vi "TDMS Logging Loop.vi"(6 "Logging Period (ms)":i64=20, 7 "Buffer Size":u32=1000, 9 "Group Initialization":T1(array[cluster]), 10 "TDMS Name":string="Test", 11 "Log to USB?":bool) -> ()   [LabVIEW 2015]
uses:
  <userlib>/836-Library/System/TDMSv2/Group Data.ctl
  <userlib>/836-Library/System/TDMSv2/Group Channels.ctl
  <vilib>/Platform/TimedLoop/XDataNode/timing_clust.ctl
  <vilib>/Platform/TimedLoop/XDataNode/nitl_modes.ctl
  <vilib>/Platform/TimedLoop/XDataNode/wakeup.ctl
  <userlib>/836-Library/System/TDMSv2/TDMS RT FIFO Packet.ctl
  <userlib>/836-Library/System/TDMSv2/Channel Initializer.ctl
  <userlib>/836-Library/System/TDMSv2/Back Channel Data.ctl
  <vilib>/platform/TimedLoop/XDataNode/XDataNode.xnode
  <vilib>/Platform/TimedLoop/XDataNode/XDNodeRunTimeDep.lvlib
panel:
  out "Cluster 2":T4
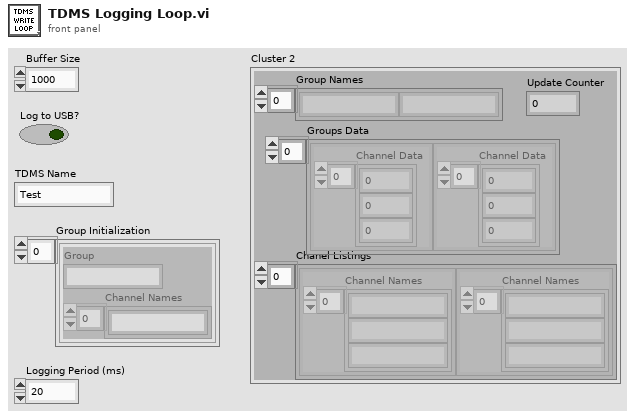
[diagram p1: front panel]
types:
  T1 = cluster{"Group":string, "Channel Names":string[]}[]
  T2 = typedef "Group Data.ctl" = cluster{"Channel Data":dbl[]}
  T3 = typedef "Group Channels.ctl" = cluster{"Channel Names":string[]}
  T4 = cluster{"Group Names":string[], "Groups Data":T2[], "Update Counter":i32, "Chanel Listings":T3[]}
  T5 = enum16{"open", "open or create", "create or replace", "create", "open (read-only)"}
  T6 = typedef "XDNodeRunTimeDep.lvlib/timing_clust.ctl" = cluster{"Expected End [f-1]":u64, "Actual End [f-1]":u64, "Finished Late? [f-1]":bool, "Expected End [i-1]":u64, "Actual End [i-1]":u64, "Finished Late? [i-1]":bool, "Expected Start [i]":u64, "Actual Start [i]":u64, "Expected Start [f]":u64, "Actual Start [f]":u64, "Source Name":string, "Structure Name":string, "Period":i64, "Deadline":i64, "Offset":i64, "Start":i64, "Priority":i32, "Timeout":i32, "Mode":T7, "Wakeup Reason":T8, "Error":errorcluster, "Source Type":string, "Secondary Source Type":string, "Global End Time":u64, "Global Start Time":u64, "Frame Duration":u64, "Iteration Duration":u64, "Assigned CPU":i32, "I/O Scan Engine Mode":u32}
  T7 = typedef "XDNodeRunTimeDep.lvlib/nitl_modes.ctl" = enum32{"No Change", "Process missed periods, maintain original phase", "Discard missed periods, maintain original phase", "Process missed periods, ignore original phase", "Discard missed periods, ignore original phase"}
  T8 = typedef "XDNodeRunTimeDep.lvlib/wakeup.ctl" = enum32{"Normal", "Aborted", "Asynchronous wakeup", "Timing source error", "Timed loop error", "Timeout"}
  T9 = typedef "Channel Initializer.ctl" = cluster{"Column Headers":string[], "Initialization array":dbl[]}
  T10 = typedef "TDMS RT FIFO Packet.ctl" = cluster{"Group/CMD":i32, "Data":dbl, "Channel":i32}
  T11 = typedef "Back Channel Data.ctl" = cluster{"Group":string, "Channel":string, "Return Notifier":refnum<notifier>}
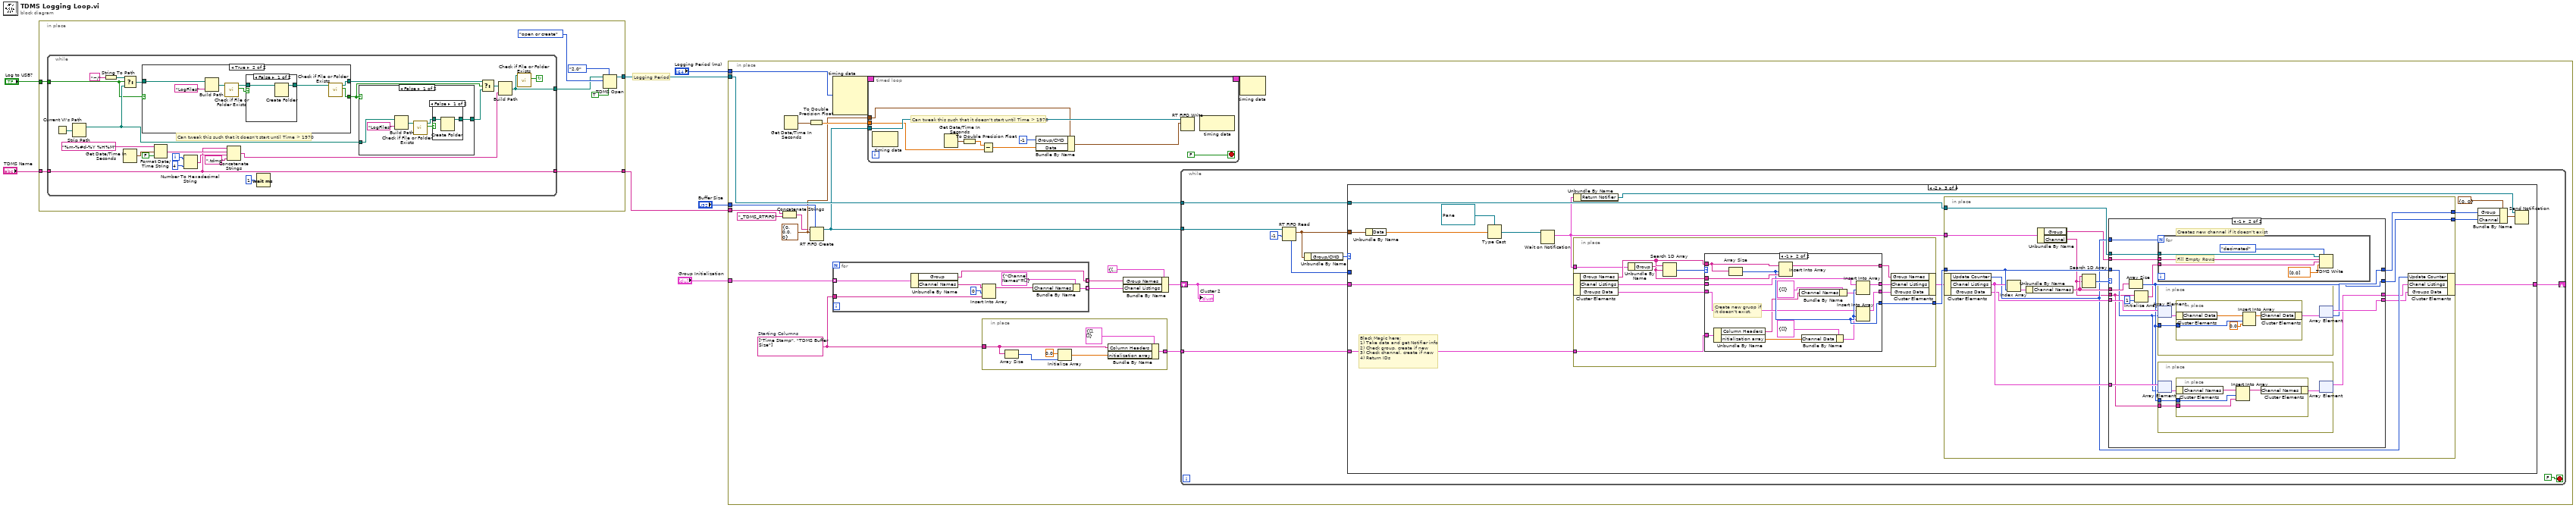
[diagram p0: block diagram]
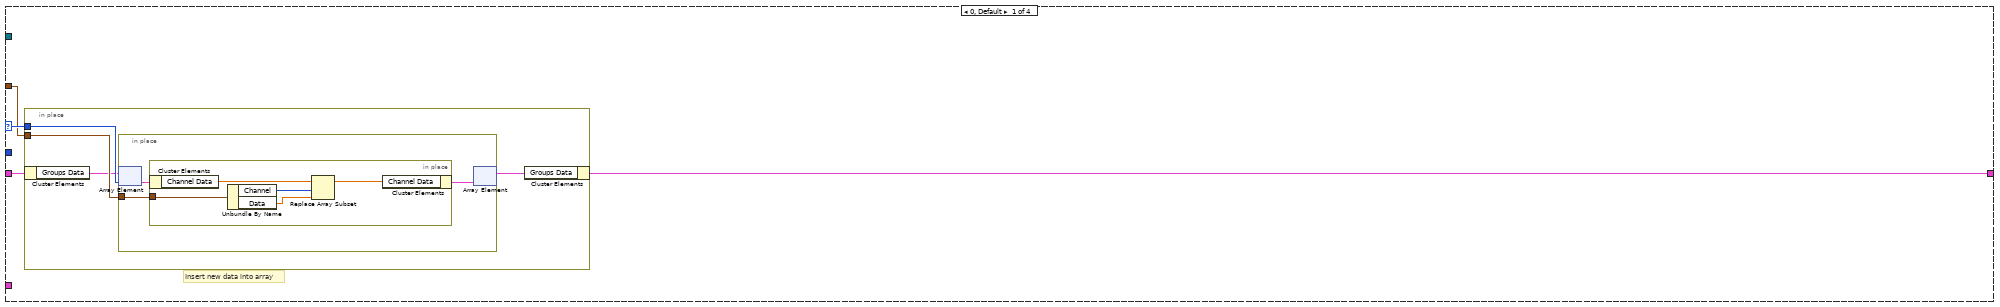
[diagram p6: hidden frame]
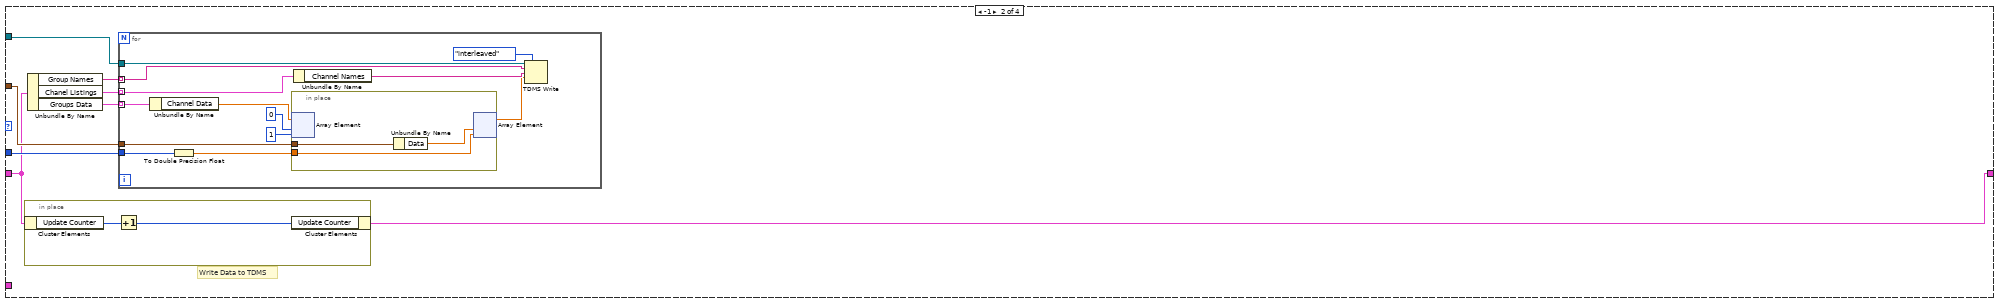
[diagram p7: hidden frame]
diagram:
  # "Logging Period"
  n1 = in-place {
    in-place-border: [w9] -> w1
    in-place-border: "Log to USB?" -> [w11]
    in-place-border: "TDMS Name" -> [w10]
    in-place-border: [w8] -> w4
    n2 = while {
      tunnel: [w28] -> w12
      tunnel: w11 -> [w17]
      tunnel: w10 -> [w16]
      tunnel: [w16] -> w8
      i -> [w32]
      stop <- w29 continue-if-true
      # "Can tweak this such that it doesn't start until Time > 1970"
      n3 = Current VI's Path() -> (path=w27:path)
      n4 = Strip Path(path=w27) -> (stripped path=w21:path)  [unwired: 1 out]
      n5 = String To Path(string="~/") -> (path=w25:path)
      n6 = Select(t=w25, s=w17, f=w21) -> (s? t:f=w26:path)
      n7 = Get Date/Time In Seconds() -> (seconds since 1Jan1904=w34:timestamp)
      n8 = case shown="True" w17 {
        selector: w17 -> [w40 _]
        tunnel: w26 -> [w39 w45]
        tunnel: [w39 w42] -> w23
        tunnel: [w40 w41] -> w20
        frame False {
        }
        frame True {
          n9 = Build Path(base path=w45, name or relative path="LogFiles") -> (appended path=w44:path)
          n10 = call <vilib>:"Check if File or Folder Exists.vi"("path"=w44) -> ("file or folder exists?"=w48:bool, "dup path"=w47:path)  [unwired: 8 in, 1 out]
          n11 = case shown="False" w48 {
            tunnel: [w50 w51] -> w43
            tunnel: w47 -> [w49 w51]
            frame False {
              n12 = Create Folder(path (use dialog)=w49) -> (created path=w50:path)  [unwired: 2 in, 2 out]
            }
            frame True {
            }
          }
          n13 = call <vilib>:"Check if File or Folder Exists.vi"("path"=w43) -> ("file or folder exists?"=w41:bool, "dup path"=w42:path)  [unwired: 8 in, 1 out]
        }
      }
      n14 = Format Date/Time String(time format string (%c)="%m-%#d-%Y %H%M", seconds (now)=w34, UTC format=FALSE) -> (date/time string=w37:string)
      n15 = Number To Hexadecimal String(1:i16 4 ("width (-)"), 2:w32) -> (0:w30:string)
      n16 = Concatenate Strings(w16, w37, w30, ".tdms" ("string")) -> (w38:string)
      n17 = Wait (ms)(milliseconds to wait=u32 1 ("millisecond multiple")) -> ()  [unwired: 1 out]
      n18 = case shown="False" w20 {
        tunnel: w21 -> [w56 w61]
        tunnel: [w52 w61] -> w19
        frame False {
          n19 = Build Path(base path=w56, name or relative path="LogFiles") -> (appended path=w53:path)
          n20 = call <vilib>:"Check if File or Folder Exists.vi"("path"=w53) -> ("file or folder exists?"=w54:bool, "dup path"=w55:path)  [unwired: 8 in, 1 out]
          n21 = case shown="False" w54 {
            tunnel: [w59 w60] -> w52
            tunnel: w55 -> [w58 w60]
            frame False {
              n22 = Create Folder(path (use dialog)=w58) -> (created path=w59:path)  [unwired: 2 in, 2 out]
            }
            frame True {
            }
          }
        }
        frame True {
        }
      }
      n23 = Select(t=w23, s=w20, f=w19) -> (s? t:f=w22:path)
      n24 = Build Path(base path=w22, name or relative path=w38) -> (appended path=w28:path)
      n25 = call <vilib>:"Check if File or Folder Exists.vi"("path"=w28) -> ("file or folder exists?"=w29:bool)  [unwired: 8 in, 2 out]
    }
    n26 = TDMS Open(6:TRUE ("disable buffering? (T)"), 7:enum16{"1.0", "2.0"}."2.0" ("file format version (2.0)"), 10:T5."open or create" ("operation (0:open)"), 11:w12) -> (3:w9:refnum<k34>)  [unwired: 3 in, 1 out]
  }
  n27 = in-place {
    in-place-border: w1 -> [w80]
    in-place-border: "Logging Period (ms)" -> [w76]
    in-place-border: w4 -> [w66]
    in-place-border: "Buffer Size" -> [w75]
    in-place-border: "Group Initialization" -> [w72]
    w67 = string[] ["Time Stamp", "TDMS Buffer Size"]  # Starting Columns
    w74 = T10 {"Group/CMD"=0, "Data"=0.0, "Channel"=0}
    n28 = Concatenate Strings(w66, "_TDMS_RTFIFO" ("string")) -> (w65:string)
    n29 = Get Date/Time In Seconds() -> (seconds since 1Jan1904=w77:timestamp)
    n30 = To Double Precision Float(number=w77) -> (double precision float=w78:dbl)
    n31 = RT FIFO Create(0:w65, 1:w74, 4:w75) -> (8:w79:refnum<k33>)  [unwired: 5 in, 2 out]
    n32 = node-c288(w76) -> (w63:T6)  [unwired: 3 in]
    n33 = for {
      tunnel: w72 -> [w103] mode=indexing
      tunnel: [w102] -> w70 mode=indexing
      tunnel: [w99] -> w68 mode=indexing
      tunnel: w67 -> [w96]
      n34 = Unbundle By Name(w103) -> ("Group"=w102:string, "Channel Names"=w101:string[])
      n35 = Insert Into Array(array=w101, index=0, new element=w96) -> (w98:string[])
      n36 = Bundle By Name(cluster=T3 {"Channel Names"=[]}, "Channel Names"=w98) -> (w99:T3)
    }
    n37 = timed-loop {
      timing: w63 -> [_]
      timing-out: [_] -> w62
      tunnel: w79 -> [w88]
      tunnel: w74 -> [w87]
      tunnel: w78 -> [w81]
      stop <- FALSE stop-if-true
      # "Can tweak this such that it doesn't start until Time > 1970"
      n38 = node-c288() -> ()  [unwired: 1 in, 1 out]
      n39 = Get Date/Time In Seconds() -> (seconds since 1Jan1904=w84:timestamp)
      n40 = To Double Precision Float(number=w84) -> (double precision float=w83:dbl)
      n41 = Subtract(x=w83, y=w81) -> (x-y=w82:dbl)
      n42 = Bundle By Name(cluster=w87, "Group/CMD"=-1 ("Index/CMD"), "Data"=w82) -> (w86:T10)
      n43 = RT FIFO Write(0:w88, 1:w86) -> ()  [unwired: 3 in, 4 out]
      n44 = node-c288() -> ()  [unwired: 1 in, 1 out]
    }
    n45 = in-place {
      in-place-border: w67 -> [w105]
      in-place-border: [w104] -> w73
      n46 = Array Size(array=w105) -> (size(s)=w108:i32)
      n47 = Initialize Array(0.0 ("element"), w108) -> (w106:dbl[])
      n48 = Bundle By Name(cluster=T9 {"Column Headers"=[], "Initialization array"=[]} ("Column Initializer"), "Column Headers"=w105, "Initialization array"=w106) -> (w104:T9)
    }
    n49 = Bundle By Name(cluster=T4 {"Group Names"=[], "Groups Data"=[], "Update Counter"=0, "Chanel Listings"=[]}, "Group Names"=w70, "Chanel Listings"=w68) -> (w69:T4)
    n50 = while {
      tunnel: w80 -> [w119]
      tunnel: w79 -> [w117]
      tunnel: w73 -> [w113]
      shift-right: [w110] -> _
      shift-left: w69 -> [w111]
      stop <- FALSE stop-if-true
      n51 = RT FIFO Read(0:w117, 2:-1 ("timeout in ms (0)")) -> (7:w115:u32, 9:w112:T10)  [unwired: 2 in, 3 out]
      n52 = Unbundle By Name(w112) -> ("Group/CMD"=w116:i32)
      n53 = case shown="-2" w116 {
        selector: w116 -> [w123 _ _ _]
        tunnel: w119 -> [_ w143 w170 _]
        tunnel: w115 -> [_ w142 _ _]
        tunnel: w113 -> [_ _ w169 _]
        tunnel: w112 -> [w122 w141 w168 _]
        tunnel: w111 -> [w121 w137 w166 w261]
        tunnel: [w120 w136 w164 w261] -> w110
        frame 0, Default {
          # "Insert new data into array"
          n54 = in-place {
            in-place-border: w123 -> [w127]
            in-place-border: w122 -> [w126]
            n55 = in-place-cluster #1(w121) -> ("Groups Data"=w125:T2[])
            n56 = in-place {
              in-place-border: w126 -> [w128]
              n57 = in-place-array #2(w125, w127) -> (w130:T2)
              n58 = in-place {
                in-place-border: w128 -> [w133]
                n59 = in-place-cluster #3(w130) -> ("Channel Data"=w135:dbl[])
                n60 = Unbundle By Name(w133) -> ("Channel"=w132:i32, "Data"=w131:dbl)
                n61 = Replace Array Subset(array=w135, new element=w131, index=w132) -> (w134:dbl[])
                n62 = in-place-cluster #3("Channel Data"=w134) -> (w129:T2)
              }
              n63 = in-place-array #2(w129) -> (w124:T2[])  [unwired: 1 out]
            }
            n64 = in-place-cluster #1("Groups Data"=w124) -> (w120:T4)
          }
        }
        frame -1 {
          # "Write Data to TDMS"
          n65 = in-place {
            n66 = in-place-cluster #4(w137) -> ("Update Counter"=w145:i32)
            n67 = Increment(x=w145) -> (x+1=w144:i32)
            n68 = in-place-cluster #4("Update Counter"=w144) -> (w136:T4)
          }
          n69 = Unbundle By Name(w137) -> ("Group Names"=w138:string[], "Chanel Listings"=w140:T3[], "Groups Data"=w139:T2[])
          n70 = for {
            tunnel: w143 -> [w158]
            tunnel: w139 -> [w157] mode=indexing
            tunnel: w140 -> [w156] mode=indexing
            tunnel: w138 -> [w155] mode=indexing
            tunnel: w142 -> [w154]
            tunnel: w141 -> [w146]
            n71 = Unbundle By Name(w157) -> ("Channel Data"=w151:dbl[])
            n72 = To Double Precision Float(number=w154) -> (double precision float=w148:dbl)
            n73 = in-place {
              in-place-border: w148 -> [w161]
              in-place-border: w146 -> [w160]
              n74 = in-place-array #5(w151, 0, 1) -> ()  [unwired: 2 out]
              n75 = Unbundle By Name(w160) -> ("Data"=w159:dbl)
              n76 = in-place-array #5(w159, w161) -> (w147:dbl[])  [unwired: 2 out]
            }
            n77 = Unbundle By Name(w156) -> ("Channel Names"=w153:string[])
            n78 = TDMS Write(0:w158, 1:enum16{"decimated", "interleaved"}."interleaved" ("data layout (0:decimated)"), 5:w155, 7:w153, 9:w147) -> ()  [unwired: 1 in, 4 out]
          }
        }
        frame -2 {
          # "Black Magic here:\n1) Take data and get Notifier info\n2) Check group, create if new\n3) Check channel, create if new\n4) Return IDs"
          n79 = Unbundle By Name(w168) -> ("Data"=w167:dbl)
          n80 = Type Cast(type=refnum<notifier> refnum ("notifier out"), x=w167) -> (*(type *) &x=w176:refnum<notifier>)
          n81 = Wait on Notification(notifier=w176) -> (notification=w162:T11)  [unwired: 3 in, 3 out]
          n82 = in-place {
            in-place-border: [w240] -> w172
            in-place-border: w169 -> [w239]
            in-place-border: w162 -> [w232]
            n83 = in-place-cluster #6(w166) -> ("Group Names"=w238:string[], "Chanel Listings"=w234:T3[], "Groups Data"=w236:T2[])
            n84 = Unbundle By Name(w232) -> ("Group"=w231:string)
            n85 = Search 1D Array(1D array=w238, element=w231) -> (index of element=w241:i32)  [unwired: 1 in]
            n86 = case shown="-1" w241 {
              selector: w241 -> [w245 _]
              tunnel: w238 -> [w244 w260]
              tunnel: w231 -> [_ w259]
              tunnel: [w245 w256] -> w240
              tunnel: [w244 w258] -> w237
              tunnel: w234 -> [w243 w257]
              tunnel: w236 -> [w242 w255]
              tunnel: [w243 w254] -> w233
              tunnel: [w242 w253] -> w235
              tunnel: w239 -> [_ w248]
              frame 0, Default {
              }
              frame -1 {
                # "Create new gruop if\nit doesn't exist."
                n87 = Unbundle By Name(w248) -> ("Column Headers"=w246:string[], "Initialization array"=w247:dbl[])
                n88 = Array Size(array=w260) -> (size(s)=w256:i32)
                n89 = Insert Into Array(array=w260, index=w256, new element=w259) -> (w258:string[])
                n90 = Bundle By Name(cluster=T3 {"Channel Names"=[]}, "Channel Names"=w246) -> (w249:T3)
                n91 = Bundle By Name(cluster=T2 {"Channel Data"=[]} ("new element/subarray"), "Channel Data"=w247) -> (w251:T2)
                n92 = Insert Into Array(array=w257, index=w256, new element=w249) -> (w254:T3[])
                n93 = Insert Into Array(array=w255, index=w256, new element=w251) -> (w253:T2[])
              }
            }
            n94 = in-place-cluster #6("Group Names"=w237, "Chanel Listings"=w233, "Groups Data"=w235) -> (w165:T4)
          }
          n95 = Unbundle By Name(w162) -> ("Return Notifier"=w163:refnum<notifier>)
          n96 = in-place {
            in-place-border: [w191] -> w173
            in-place-border: w172 -> [w188]
            in-place-border: [w187] -> w171
            in-place-border: w170 -> [w186]
            in-place-border: w162 -> [w180]
            n97 = in-place-cluster #7(w165) -> ("Update Counter"=w183:i32, "Chanel Listings"=w185:T3[], "Groups Data"=w184:T2[])
            n98 = Index Array(array=w185, index=w188) -> (element=w190:T3)
            n99 = Unbundle By Name(w190) -> ("Channel Names"=w189:string[])
            n100 = Unbundle By Name(w180) -> ("Group"=w178:string, "Channel"=w179:string)
            n101 = Search 1D Array(1D array=w189, element=w179) -> (index of element=w192:i32)  [unwired: 1 in]
            n102 = case shown="-1" w192 {
              selector: w192 -> [w195 _]
              tunnel: [w196 w204] -> w182
              tunnel: w185 -> [w196 w206]
              tunnel: [w195 w205] -> w191
              tunnel: [w194 w208] -> w181
              tunnel: w184 -> [w194 w209]
              tunnel: w189 -> [_ w210]
              tunnel: w188 -> [w193 w203]
              tunnel: [w193 w207] -> w187
              tunnel: w179 -> [_ w199]
              tunnel: w183 -> [_ w202]
              tunnel: w178 -> [_ w201]
              tunnel: w186 -> [_ w197]
              frame 0, Default {
              }
              frame -1 {
                # "Creates new channel if it doesn't exist"
                n103 = Array Size(array=w210) -> (size(s)=w205:i32)
                n104 = Initialize Array(w199, 1 ("dimension size")) -> (w198:string[])
                n105 = for {
                  N: w202 -> [_]
                  tunnel: w201 -> [w214]
                  tunnel: w198 -> [w213]
                  tunnel: w197 -> [w211]
                  # "Fill Empty Rows"
                  n106 = TDMS Write(0:w211, 1:enum16{"decimated", "interleaved"}."decimated" ("data layout (0:decimated)"), 5:w214, 7:w213, 9:dbl[] [0.0]) -> ()  [unwired: 1 in, 4 out]
                }
                n107 = in-place {
                  in-place-border: w205 -> [w224]
                  n108 = in-place-array #8(w209, w203) -> (w226:T2)
                  n109 = in-place {
                    in-place-border: w224 -> [w229]
                    n110 = in-place-cluster #9(w226) -> ("Channel Data"=w230:dbl[])
                    n111 = Insert Into Array(array=w230, index=w229, new element=0.0 ("new element/subarray")) -> (w227:dbl[])
                    n112 = in-place-cluster #9("Channel Data"=w227) -> (w225:T2)
                  }
                  n113 = in-place-array #8(w225) -> (w208:T2[], w207:i32)
                }
                n114 = in-place {
                  in-place-border: w205 -> [w217]
                  in-place-border: w199 -> [w216]
                  n115 = in-place-array #10(w206, w203) -> (w219:T3)
                  n116 = in-place {
                    in-place-border: w217 -> [w222]
                    in-place-border: w216 -> [w220]
                    n117 = in-place-cluster #11(w219) -> ("Channel Names"=w223:string[])
                    n118 = Insert Into Array(array=w223, index=w222, new element=w220) -> (w221:string[])
                    n119 = in-place-cluster #11("Channel Names"=w221) -> (w218:T3)
                  }
                  n120 = in-place-array #10(w218) -> (w204:T3[])  [unwired: 1 out]
                }
              }
            }
            n121 = in-place-cluster #7("Update Counter"=w183, "Chanel Listings"=w182, "Groups Data"=w181) -> (w164:T4)
          }
          n122 = Bundle By Name(cluster=cluster{"Group":i32, "Channel":i32} {"Group"=0, "Channel"=0} ("notification"), "Group"=w171, "Channel"=w173) -> (w174:cluster{"Group":i32, "Channel":i32})
          n123 = Send Notification(notification=w174, notifier=w163) -> ()  [unwired: 1 in, 2 out]
        }
        frame -3 {
          # "Do Nothing"
        }
      }
      "Cluster 2" <- w111
    }
    n124 = node-c288(w62) -> ()  [unwired: 1 out]
  }
